vi "Case.vi"   [LabVIEW 2017]
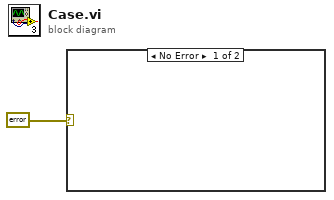
[diagram p0: block diagram]
diagram:
  n1 = case shown="No Error" errorcluster {"status"=FALSE, "code"=0, "source"=""} ("error IO") {
    frame No Error {
    }
    frame Error {
    }
  }
